vi "xml_builder.vi"(7 "parameters":T1[](array[typedef]), 8 "error in (no error)":errorcluster, 10 "content":string, 11 "tag":string) -> (0 "error out":errorcluster, 3 "xml string":string)   [LabVIEW 2010]
uses:
  clusters/key_value_cluster.ctl
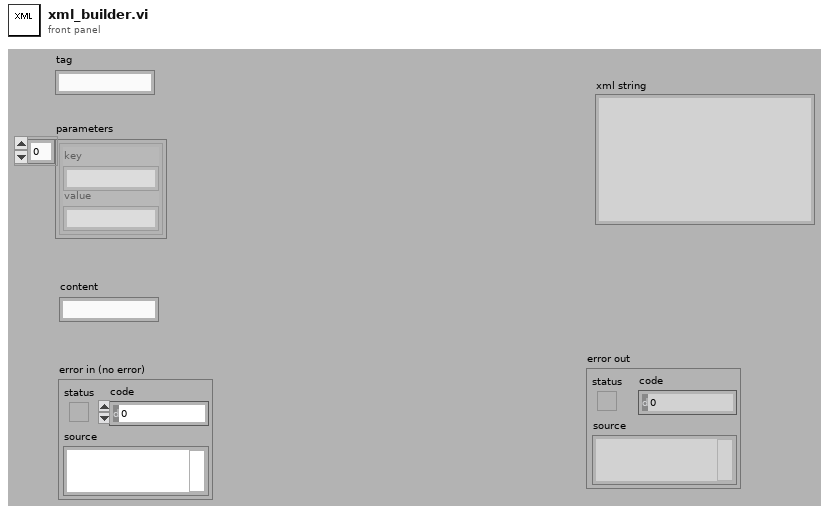
[diagram p1: front panel]
types:
  T1 = typedef "key_value_cluster.ctl" = cluster{"key":string, "value":string}
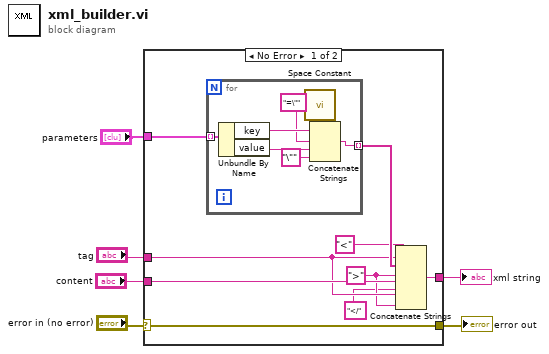
[diagram p0: block diagram]
diagram:
  n1 = case shown="No Error" "error in (no error)" {
    selector: "error in (no error)" -> [w9 w23]
    tunnel: "parameters" -> [w15 _]
    tunnel: "content" -> [w13 _]
    tunnel: "tag" -> [w11 _]
    tunnel: [w10 _] -> w3
    tunnel: [w9 w23] -> w1
    frame No Error {
      w8 = ">"
      n2 = for {
        tunnel: w15 -> [w22] mode=indexing
        tunnel: [w17] -> w14 mode=indexing
        n3 = Unbundle By Name(w22) -> ("key"=w21:string, "value"=w19:string)
        n4 = call <vilib>:"Space Constant.vi"() -> ("String"=w16:string)
        n5 = Concatenate Strings(w16, w21, "=\"", w19, "\"" ("string")) -> (w17:string)
      }
      n6 = Concatenate Strings("<", w11, w14, w8, w13, "</" ("string"), w11, w8) -> (w10:string)
    }
    frame Error {
    }
  }
  "xml string" <- w3
  "error out" <- w1
